vi "Open Test Case.vi"(8 "error in (no error)":errorcluster, 10 "Tag":string, 11 "Open Test Case in":refnum<class "Open Test Case.lvclass">) -> (0 "error out":errorcluster, 1 "VI name valid?":bool, 3 "Open Test Case out":refnum<class "Open Test Case.lvclass">)   [LabVIEW 2020, in "Open Test Case.lvclass"]
uses:
  Open Test Case.lvclass
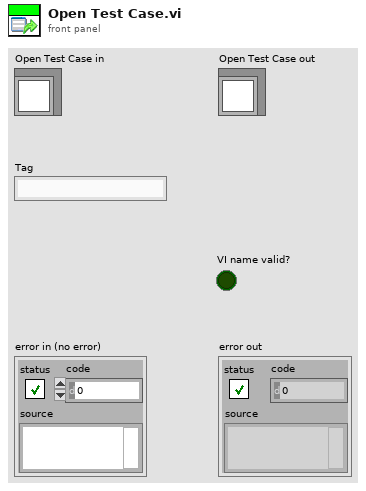
[diagram p1: front panel]
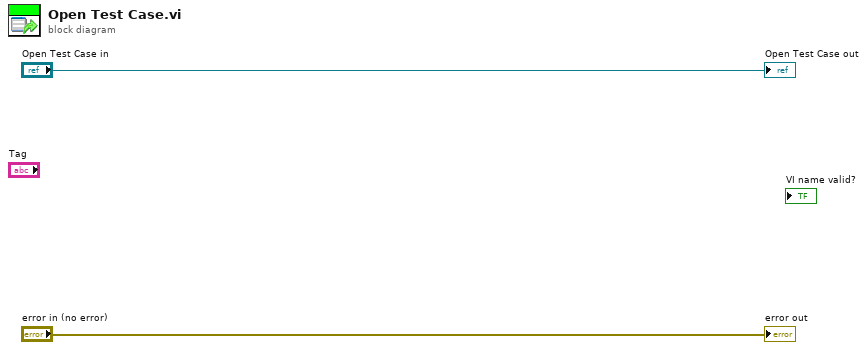
[diagram p0: block diagram]
diagram:
  "error out" <- "error in (no error)"
  "Open Test Case out" <- "Open Test Case in"
